vi "SPC_save_FifoImage_to_sdtfile.vi"(5 "SdtInfo":T1={"imageSize"=2, "module_no"=2, "module_type"=2, "adc_resolution][exp]"=2, "NumRoutingCh"=2, "serial_no"=""}, 6 "SDTFilename":path, 7 "SPCdata In":T2={"base_adr"=896, "init"=0, "cfd_limit_low"=5.0, "cfd_limit_high"=80.0, "cfd_zc_level"=0.0, "cfd_holdoff"=5.0, "sync_zc_level"=0.0, "sync_holdoff"=4.0, "sync_threshold"=-20.0, "tac_range"=50.0, "sync_freq_div"=1, "tac_gain"=1, "tac_offset"=0.0, "tac_limit_low"=10.0, "tac_limit_high"=80.0, "adc_resolution"=10, "ext_latch_delay"=0, "collect_time"=0.01, "display_time"=1.0, "repeat_time"=10.0001, "stop_on_time"=1, "stop_on_ovfl"=1, "dither_range"=0, "count_incr"=1, "mem_bank"=0, "dead_time_comp"=1, "scan_control"=61440, "routing_mode"=0, "tac_enable_hold"=10.0, "pci_card_no"=-1, "mode"=0, "scan_size_x"=1, "scan_size_y"=1, "scan_rout_x"=1, "scan_rout_y"=1, "scan_flyback"=0, "scan_borders"=0, "scan_polarity"=0, "pixel_clock"=0, "line_compression"=1, "trigger"=0, "pixel_time"=5e-08, "ext_pixclk_div"=1, "rate_count_time"=1.0, "macro_time_clk"=0, "add_select"=0, "test_eep"=0, "adc_zoom"=0, "img_size_x"=1, "img_size_y"=1, "img_rout_x"=1, "img_rout_y"=1, "xy_gain"=1, "master_clock"=0, "adc_sample_delay"=0, "detector_type"=1, "chan_enable"=4191231, "chan_slope"=0, "chan_spec_no"=34835, "tdc_control"=0, "tdc_offset1"=0.0, "tdc_offset2"=0.0, "tdc_offset3"=0.0, "tdc_offset4"=0.0, "future_reserve1"=0, "future_reserve2"=0, "future_reserve3"=0, "future_reserve4"=0, "future_reserve5"=0, "future_reserve6"=0, "future_reserve7"=0}, 8 "Error In":errorcluster, 9 "FifoImageData":u16[](array[numeric]), 11 "DLL Path":path) -> (0 "Error Out":errorcluster, 3 "DLL Path":path)   [LabVIEW 2019]
doc: "The procedure sends all parameters from the ‘SPCdata’ structure to the internal DLL structures of the module ‘mod_no’ and to the control registers of the SPC module ‘mod_no’.\nThe new parameter values are recalculated according to the parameter limits, hardware restrictions (e.g. DAC resolution) and the SPC module type. Furthermore, cross dependencies between different parameters are taken into account to ensure the correct hardware operation. \nThis VI also calls SPC_get_parameters after the call to SPC_set_parameters to provide the actual values after recalculation.\nIf an error occurs at a particular parameter, the procedure does not set the rest of the parameters and returns with an error code\n\ninfo@becker-hickl.com"
uses:
  SPC_Controls/SPCdata.ctl
  SPC_Controls/SdtInfoJannis.ctl
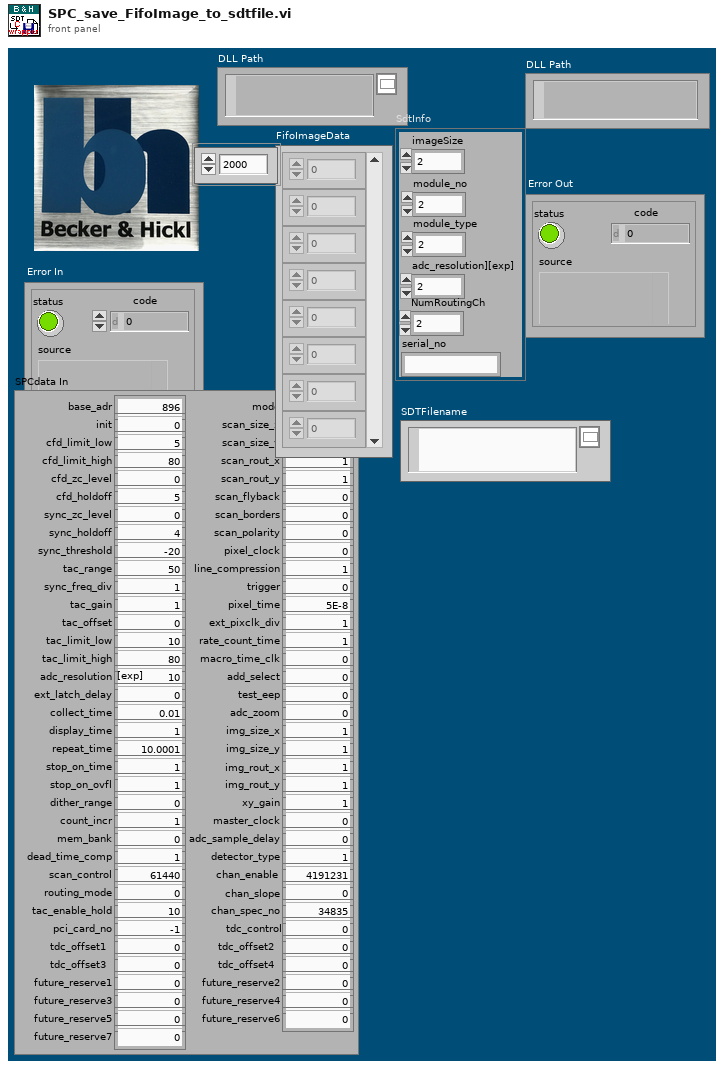
[diagram p1: front panel]
types:
  T1 = typedef "SdtInfoJannis.ctl" = cluster{"imageSize":i32, "module_no":i16, "module_type":i16, "adc_resolution][exp]":i16, "NumRoutingCh":u16, "serial_no":string}
  T2 = typedef "SPCdata.ctl" = cluster{"base_adr":u16, "init":i16, "cfd_limit_low":sgl, "cfd_limit_high":sgl, "cfd_zc_level":sgl, "cfd_holdoff":sgl, "sync_zc_level":sgl, "sync_holdoff":sgl, "sync_threshold":sgl, "tac_range":sgl, "sync_freq_div":i16, "tac_gain":i16, "tac_offset":sgl, "tac_limit_low":sgl, "tac_limit_high":sgl, "adc_resolution":i16, "ext_latch_delay":i16, "collect_time":sgl, "display_time":sgl, "repeat_time":sgl, "stop_on_time":i16, "stop_on_ovfl":i16, "dither_range":i16, "count_incr":i16, "mem_bank":i16, "dead_time_comp":i16, "scan_control":u16, "routing_mode":u16, "tac_enable_hold":sgl, "pci_card_no":i16, "mode":u16, "scan_size_x":u32, "scan_size_y":u32, "scan_rout_x":u32, "scan_rout_y":u32, "scan_flyback":u32, "scan_borders":u32, "scan_polarity":u16, "pixel_clock":u16, "line_compression":u16, "trigger":u16, "pixel_time":sgl, "ext_pixclk_div":u32, "rate_count_time":sgl, "macro_time_clk":i16, "add_select":i16, "test_eep":i16, "adc_zoom":i16, "img_size_x":u32, "img_size_y":u32, "img_rout_x":u32, "img_rout_y":u32, "xy_gain":i16, "master_clock":i16, "adc_sample_delay":i16, "detector_type":i16, "chan_enable":u32, "chan_slope":u32, "chan_spec_no":u32, "tdc_control":u32, "tdc_offset1":sgl, "tdc_offset2":sgl, "tdc_offset3":sgl, "tdc_offset4":sgl, "future_reserve1":u64, "future_reserve2":u64, "future_reserve3":u64, "future_reserve4":u64, "future_reserve5":u64, "future_reserve6":u64, "future_reserve7":u64}
  T3 = cluster{"imageSize":i32, "module_no":i16, "module_type":i16, "adc_resolution][exp]":i16, "NumRoutingCh":u16, u8, u8, u8, u8, u8, u8, u8, u8, u8, u8, u8, u8, u8, u8, u8, u8}
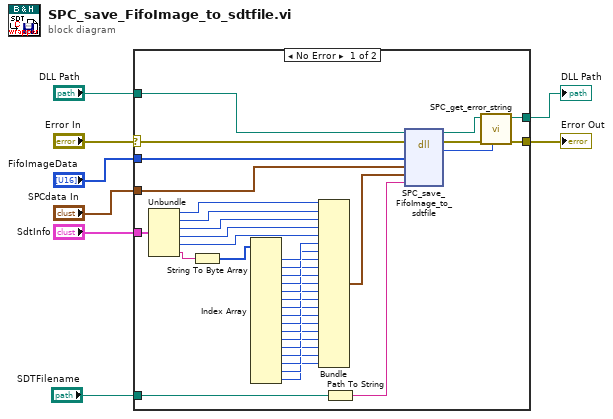
[diagram p0: block diagram]
diagram:
  n1 = case shown="No Error" "Error In" {
    selector: "Error In" -> [w43 w45]
    tunnel: "DLL Path" -> [w44 w46]
    tunnel: [w34 w45] -> w7
    tunnel: [w39 w46] -> w6
    tunnel: "SPCdata In" -> [w42 _]
    tunnel: "SDTFilename" -> [w36 _]
    tunnel: "FifoImageData" -> [w35 _]
    tunnel: "SdtInfo" -> [w33 _]
    frame No Error {
      n2 = Unbundle(w33) -> ("imageSize"=w15:i32, "module_no"=w14:i16, "module_type"=w13:i16, "adc_resolution][exp]"=w12:i16, "NumRoutingCh"=w10:u16, "serial_no"=w9:string)
      n3 = String To Byte Array(string=w9) -> (unsigned byte array=w11:u8[])
      n4 = Index Array(array=w11) -> (element #1=w31:u8, element #2=w30:u8, element #3=w29:u8, element #4=w28:u8, element #5=w27:u8, element #6=w26:u8, element #7=w25:u8, element #8=w24:u8, element #9=w23:u8, element #10=w22:u8, element #11=w21:u8, element #12=w20:u8, element #13=w19:u8, element #14=w18:u8, element #15=w17:u8, element #16=w16:u8)  [unwired: 16 in]
      n5 = Bundle("imageSize"=w15, "module_no"=w14, "module_type"=w13, "adc_resolution][exp]"=w12, "NumRoutingCh"=w10, w31, w30, w29, w28, w27, w26, w25, w24, w23, w22, w21, w20, w19, w18, w17, w16) -> (w32:T3)  [unwired: 1 in]
      n6 = Path To String(path=w36) -> (string=w37:string)
      n7 = dll-call lib="D:/spcm/lib/lab_view/lv10.0/spcm32.dll" fn="SPC_save_FifoImage_to_sdtfile"(path in=w44, error in=w43, "data_buf"=w35, "SPCdata"=w42, "SdtInfo"=w32, "sdt_file"=w37) -> (path out=w38:path, error out=w40:errorcluster, "return type"=w41:i16)  [unwired: 5 in]
      n8 = call "SPC_get_error_string.vi"("ErrorID"=w41, "Error In"=w40, "DLL Path"=w38) -> ("Error Out"=w34:errorcluster, "DLL Path"=w39:path)  [unwired: 6 in, 1 out]
    }
    frame Error {
    }
  }
  "DLL Path" <- w6
  "Error Out" <- w7
